vi "picoquant_set_sync.vi"(8 "error in (no error)":errorcluster, 10 "Sync Settings":T1 {"snc_offs" min=-99999 max=99999 step=1; "snc_ZeroX" min=0 max=20 step=1; "snc_level" min=0 max=800 step=10}, 11 "picoquant_generic in":refnum<class "picoquant_generic.lvclass">) -> (0 "error out":errorcluster, 3 "picoquant_generic out":refnum<class "picoquant_generic.lvclass">)   [LabVIEW 2015, in "picoquant_generic.lvclass"]
uses:
  picoquant_generic.lvclass
  Hydraharp/hydraharp_panel/hpanel_sync_settings.ctl
  Hydraharp/hydraharp_panel/hpanel_sync_div.ctl
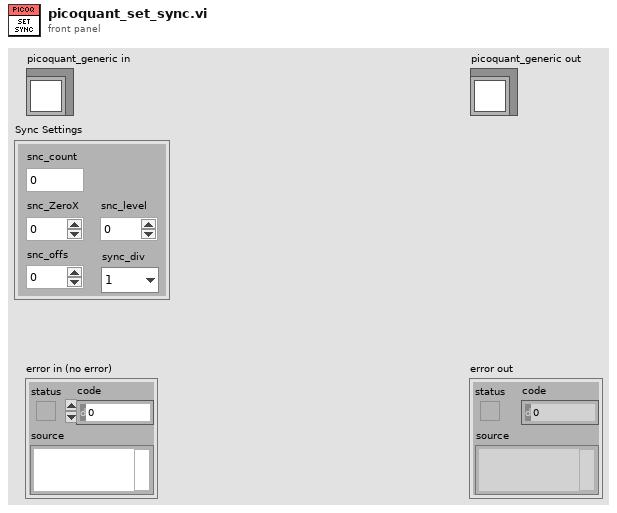
[diagram p1: front panel]
types:
  T1 = typedef "hpanel_sync_settings.ctl" = cluster{"snc_count":i32, "snc_level":i32, "snc_ZeroX":i32, "snc_offs":i32, "sync_div":T2}
  T2 = typedef "hpanel_sync_div.ctl" = enum16{"1", "2", "4", "8"}
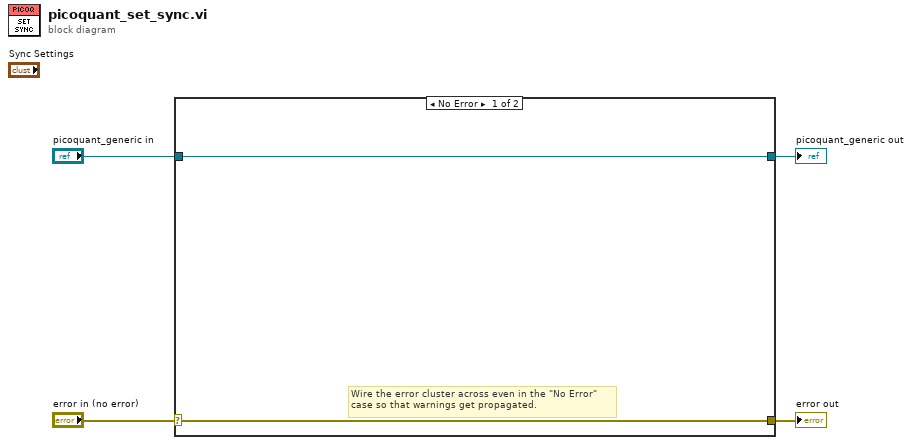
[diagram p0: block diagram]
diagram:
  n1 = case shown="No Error" "error in (no error)" {
    selector: "error in (no error)" -> [w5 w8]
    tunnel: [w5 w8] -> w3
    tunnel: [w6 w7] -> w1
    tunnel: "picoquant_generic in" -> [w6 w7]
    frame No Error {
      # "Wire the error cluster across even in the \"No Error\"\ncase so that warnings get propagated."
    }
    frame Error {
    }
  }
  "error out" <- w3
  "picoquant_generic out" <- w1
